vi "Pause_for_server_ch_val.vi"(2 "Extra command string":string, 3 "Simulate/Run":T1) -> (0 "Extra command string Out":string, 1 "Error Comments":string)   [LabVIEW 2010]
uses:
  Controls/User_Specific_mode.ctl
  ADAM Client/Sub VIs/ADAM Controls/Channel_names.ctl
  Globals/Extra_Commands_Global.vi
panel:
  out "Minutes Waited":dbl format="%.2f"
  out "Channel Found?":bool
  out "Time to email next":dbl format="%.2f"
  out "Actual Value":string
  out "Channel Value":string
  out "Channel Name":string
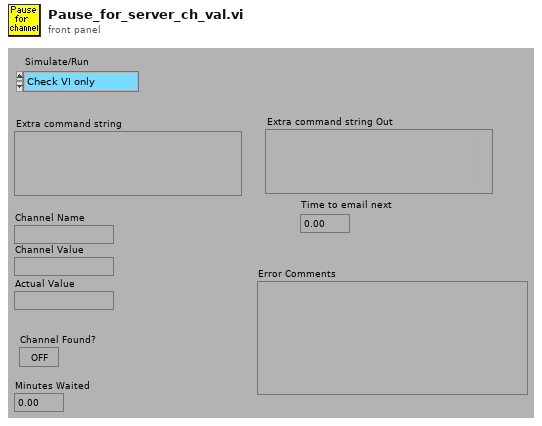
[diagram p1: front panel]
types:
  T1 = typedef "User_Specific_mode.ctl" = enum16{"Check VI only", "Run VI"}
  T2 = typedef "Channel_names.ctl" = enum16{"Active Only", "Active + Off", "All Channels"}
  T3 = typedef "Ch_description_ADAM.ctl" = cluster{"Ch Name":string, "Type":T4, "Function":T5, "Ch State":T6, "Calibration type":T7, "A":dbl, "B":dbl, "C":dbl, "D":dbl, "Comments":string, "Address":T8, "String":string, "Duty":u16}
  T4 = typedef "Module_type_ADAM.ctl" = enum16{"4011", "4012", "4013", "4014", "4016", "4017", "4018", "4021", "4050", "4052", "4053", "4060", "4080", "5000", "5017", "5018", "5024", "5051", "5056", "5060", "6060", "Tracker", "WEST", "GILL", "JEM", "VICI", "Vaisala", "DRUCK", "Run VI Named:", "IR2100", "PPT", "Comparator", "VIRTUAL", "Hold Value", "Read A", "Read Ch", "Coded", "Client Info", "Web Client", "X10", "Test"}
  T5 = typedef "Function_ADAM.ctl" = enum16{"Analogue Input", "Digital Input", "Event counter", "Event rate", "Analogue Output", "Digital Output", "Relay Output"}
  T6 = typedef "Channel_State.ctl" = enum16{"On", "Off", "Always On", "Always Off"}
  T7 = typedef "Calib_type_ADAM.ctl" = enum16{"Raw", "Bx + A", "Cx^2 + Bx + A", "Dx^3 + Cx^2 + Bx + A", "In Band", "Hi-Tec Q", "Hi-Tec M_dot", "Text"}
  T8 = typedef "Address.ctl" = cluster{"Main":i32, "Ch.":i32, "Sub":i32, "Port Name":string}
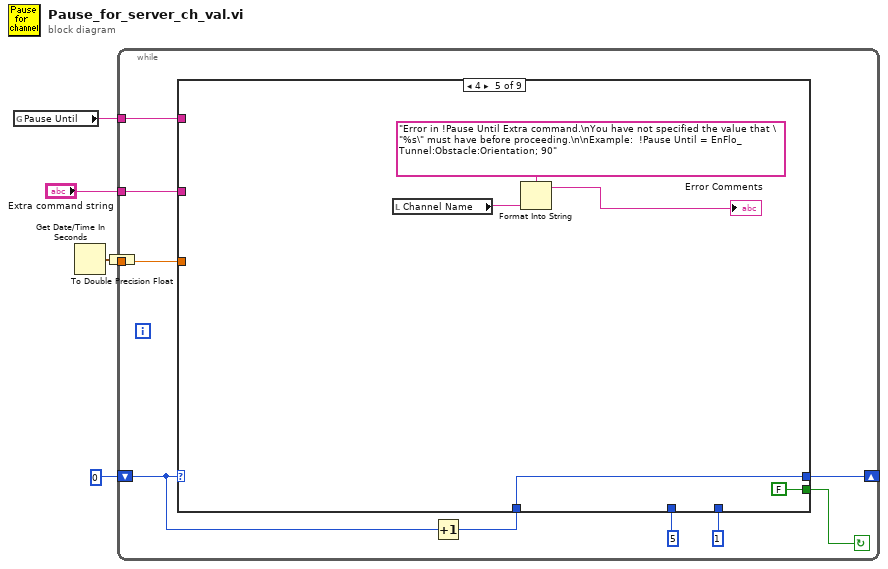
[diagram p0: block diagram]
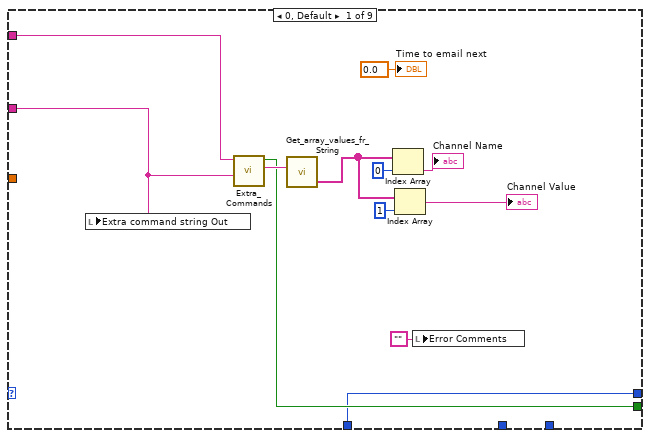
[diagram p2: hidden frame]
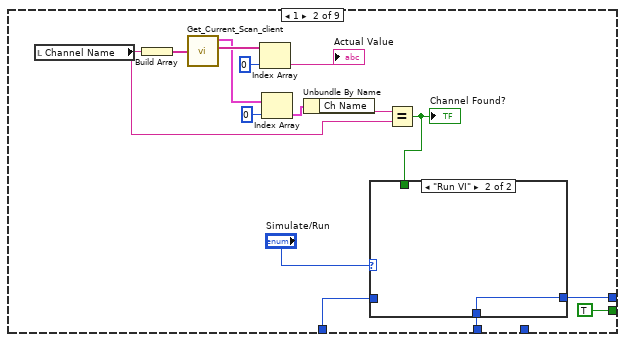
[diagram p3: hidden frame]
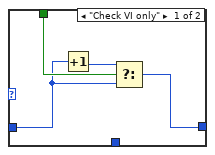
[diagram p4: hidden frame]
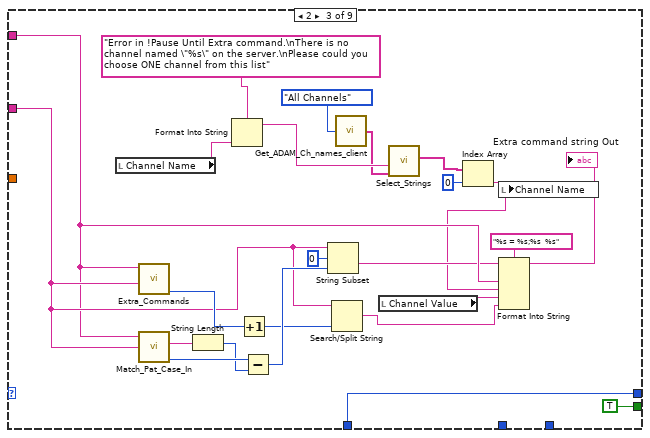
[diagram p5: hidden frame]
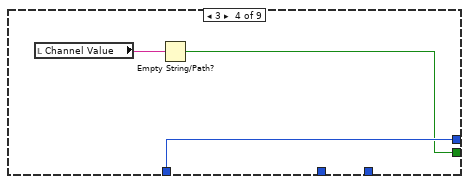
[diagram p6: hidden frame]
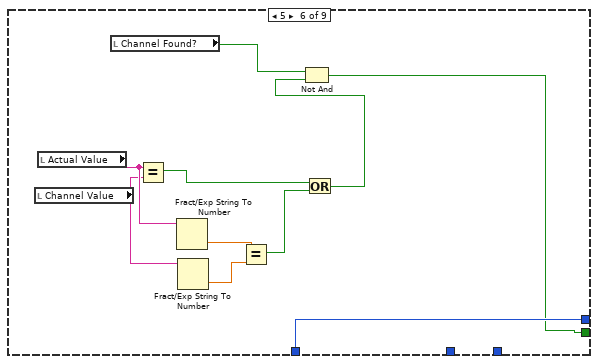
[diagram p7: hidden frame]
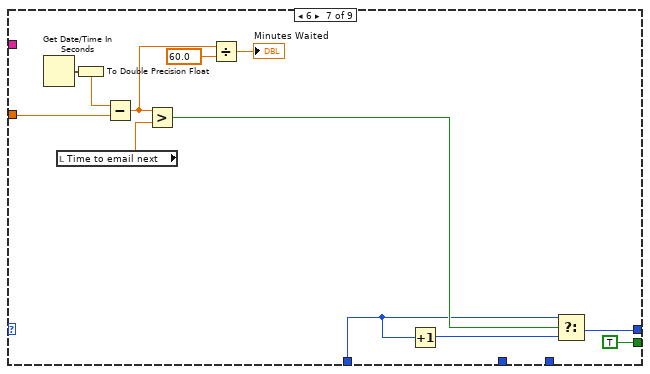
[diagram p8: hidden frame]
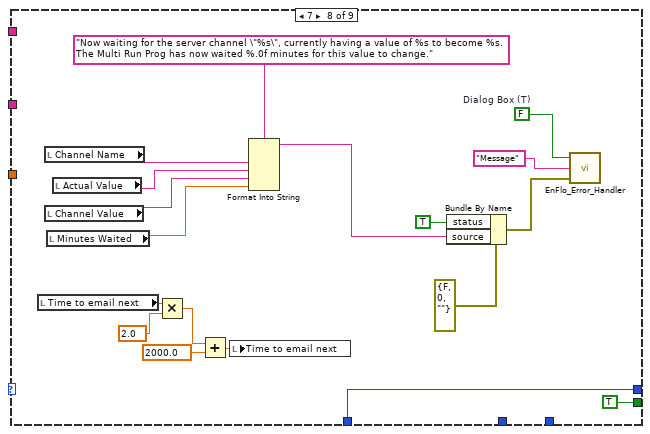
[diagram p9: hidden frame]
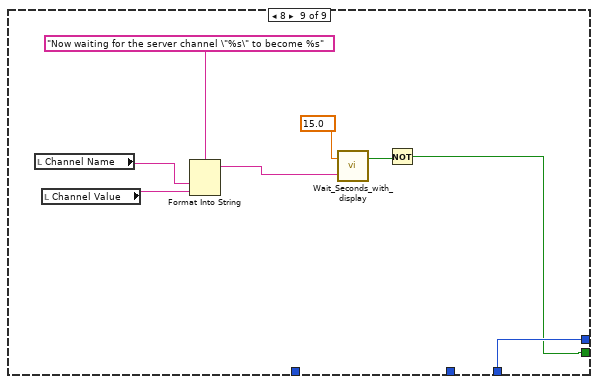
[diagram p10: hidden frame]
diagram:
  n1 = global read "Extra_Commands_Global.vi" "Pause Until"() -> (w3:string)
  n2 = Get Date/Time In Seconds() -> (seconds since 1Jan1904=w1:timestamp)
  n3 = To Double Precision Float(number=w1) -> (double precision float=w2:dbl)
  n4 = while {
    tunnel: w2 -> [w7]
    tunnel: w3 -> [w8]
    tunnel: "Extra command string" -> [w9]
    shift-left: 0 -> [w13]
    shift-right: [w11] -> _
    stop <- w14 continue-if-true
    n5 = Increment(x=w13) -> (x+1=w12:i32)
    n6 = case shown="4" w13 {
      tunnel: [w21 TRUE ("Command Found") TRUE ("Command Found") w71 FALSE ("Command Found") w86 TRUE ("Command Found") TRUE ("Command Found") w119] -> w14
      tunnel: w12 -> [w20 w30 w50 w73 w78 w88 w95 w118 _]
      tunnel: [w20 w29 w50 w73 w78 w88 w93 w118 w121] -> w11
      tunnel: 5 ("f") -> [_ w28 _ _ _ _ _ _ _]
      tunnel: w9 -> [w17 _ w57 _ _ _ _ _ _]
      tunnel: w8 -> [w18 _ w56 _ _ _ _ _ _]
      tunnel: w7 -> [_ _ _ _ _ _ w97 _ _]
      tunnel: 1 ("f") -> [_ _ _ _ _ _ _ _ w121]
      frame 0, Default {
        n7 = local write "Extra command string Out"(w17) -> ()
        n8 = call "Extra_Commands.vi"("String to Search"=w17, "Command"=w18) -> ("String Value"=w26:string, "Command Found"=w21:bool)  [unwired: 1 in, 3 out]
        n9 = call "Get_array_values_fr_String.vi"("String Value"=w26) -> ("String array"=w23:string[])  [unwired: 1 out]
        n10 = Index Array(array=w23, index=0 ("Index")) -> (element=→"Channel Name":string)
        n11 = Index Array(array=w23, index=1 ("Index")) -> (element=→"Channel Value":string)
        n12 = local write "Error Comments"("") -> ()
        "Time to email next" <- 0.0 ("Time to email next")
      }
      frame 1 {
        n13 = local read "Channel Name"() -> (w33:string)
        n14 = Build Array(w33) -> (w41:string[])
        n15 = call "Get_Current_Scan_client.vi"("ADAM Ch Names"=w41) -> ("Ch Description Array"=w37:T3[], "String values"=w40:string[])  [unwired: 2 out]
        n16 = Index Array(array=w40, index=0 ("Index")) -> (element=→"Actual Value":string)
        n17 = Index Array(array=w37, index=0 ("Index")) -> (element=w36:T3)
        n18 = Unbundle By Name(w36) -> ("Ch Name"=w35:string)
        n19 = Equal?(x=w35, y=w33) -> (x = y?=w27:bool)
        "Channel Found?" <- w27
        n20 = case shown="\"Run VI\"" "Simulate/Run" {
          tunnel: w30 -> [w43 _]
          tunnel: [w42 w46] -> w29
          tunnel: w28 -> [_ w46]
          tunnel: w27 -> [w45 _]
          frame "Check VI only" {
            n21 = Increment(x=w43) -> (x+1=w44:i32)
            n22 = Select(t=w44, s=w45, f=w43) -> (s? t:f=w42:i32)
          }
          frame "Run VI" {
          }
        }
      }
      frame 2 {
        n23 = local read "Channel Name"() -> (w68:string)
        n24 = call "Extra_Commands.vi"("String to Search"=w57, "Command"=w56) -> ("Offset Past Command"=w58:i32)  [unwired: 1 in, 4 out]
        n25 = call "Match_Pat_Case_In.vi"("String to match"=w56, "String"=w57) -> ("Matched string"=w63:string, "offset past match"=w62:i32)  [unwired: 1 in, 2 out]
        n26 = String Length(string=w63) -> (length=w61:i32)
        n27 = Format Into String(format string="Error in !Pause Until Extra command.\nThere is no channel named \"%s\" on the server.\nPlease could you choose ONE channel from this list" ("Format String"), w68) -> (resulting string=w67:string)  [unwired: 2 in, 1 out]
        n28 = Increment(x=w58) -> (x+1=w48:i32)
        n29 = Subtract(x=w62, y=w61) -> (x-y=w60:i32)
        n30 = String Subset(string=w57, offset (0)=0, length (rest)=w60) -> (substring=w55:string)
        n31 = Search/Split String(string=w57, offset (0)=w48) -> (match + rest of string=w54:string)  [unwired: 3 out]
        n32 = call "Get_ADAM_Ch_names_client.vi"("Channel names set"=Channel_names."All Channels") -> ("Ch names"=w65:string[])
        n33 = local read "Channel Value"() -> (w51:string)
        n34 = call "Select_Strings.vi"("Available Ch names"=w65, "Message"=w67) -> ("Selected Channel Names"=w47:string[])  [unwired: 2 in, 4 out]
        n35 = Index Array(array=w47, index=0 ("Index")) -> (element=w49:string)
        n36 = local write "Channel Name"(w49) -> ()
        n37 = Format Into String(format string="%s = %s;%s  %s" ("Format String"), initial string=w55, w56, w49, w51, w54) -> (resulting string=→"Extra command string Out":string)  [unwired: 1 in, 1 out]
      }
      frame 3 {
        n38 = local read "Channel Value"() -> (w72:string)
        n39 = Empty String/Path?(string/path=w72) -> (empty?=w71:bool)
      }
      frame 4 {
        n40 = local read "Channel Name"() -> (w74:string)
        n41 = Format Into String(format string="Error in !Pause Until Extra command.\nYou have not specified the value that \"%s\" must have before proceeding.\n\nExample:  !Pause Until = EnFlo_Tunnel:Obstacle:Orientation; 90", w74) -> (resulting string=→"Error Comments":string)  [unwired: 2 in, 1 out]
      }
      frame 5 {
        n42 = local read "Channel Value"() -> (w84:string)
        n43 = local read "Actual Value"() -> (w85:string)
        n44 = local read "Channel Found?"() -> (w87:bool)
        n45 = Equal?(x=w85, y=w84) -> (x = y?=w81:bool)
        n46 = Fract/Exp String To Number(string=w85) -> (number=w83:dbl)  [unwired: 4 out]
        n47 = Fract/Exp String To Number(string=w84) -> (number=w82:dbl)  [unwired: 4 out]
        n48 = Equal?(x=w83, y=w82) -> (x = y?=w80:bool)
        n49 = Or(x=w81, y=w80) -> (x .or. y?=w79:bool)
        n50 = Not And(1:w79, 2:w87) -> (0:w86:bool)
      }
      frame 6 {
        n51 = Get Date/Time In Seconds() -> (seconds since 1Jan1904=w89:timestamp)
        n52 = local read "Time to email next"() -> (w98:dbl)
        n53 = To Double Precision Float(number=w89) -> (double precision float=w99:dbl)
        n54 = Subtract(x=w99, y=w97) -> (x-y=w92:dbl)
        n55 = Greater?(x=w92, y=w98) -> (0:w96:bool)
        n56 = Divide(x=w92, y=60.0) -> (x/y=→"Minutes Waited":dbl)
        n57 = Increment(x=w95) -> (x+1=w94:i32)
        n58 = Select(t=w95, s=w96, f=w94) -> (s? t:f=w93:i32)
      }
      frame 7 {
        w114 = FALSE  # Dialog Box (T)
        n59 = local read "Time to email next"() -> (w105:dbl)
        n60 = local read "Channel Name"() -> (w113:string)
        n61 = local read "Channel Value"() -> (w111:string)
        n62 = local read "Minutes Waited"() -> (w110:dbl)
        n63 = local read "Actual Value"() -> (w112:string)
        n64 = Multiply(x=w105, y=2.0) -> (x*y=w103:dbl)
        n65 = Add(x=w103, y=2000.0) -> (x+y=w101:dbl)
        n66 = local write "Time to email next"(w101) -> ()
        n67 = Format Into String(format string="Now waiting for the server channel \"%s\", currently having a value of %s to become %s. The Multi Run Prog has now waited %.0f minutes for this value to change." ("Format String"), w113, w112, w111, w110) -> (resulting string=w106:string)  [unwired: 2 in, 1 out]
        n68 = Bundle By Name(cluster=errorcluster {"status"=FALSE, "code"=0, "source"=""} ("error in (no error)"), "status"=TRUE ("Bundle Element"), "source"=w106) -> (w115:errorcluster)
        n69 = call "EnFlo_Error_Handler.vi"("error in (no error)"=w115, "Error Type"="Message", "Dialog Box (T)"=w114) -> ()  [unwired: 3 out]
      }
      frame 8 {
        n70 = local read "Channel Name"() -> (w125:string)
        n71 = local read "Channel Value"() -> (w124:string)
        n72 = Format Into String(format string="Now waiting for the server channel \"%s\" to become %s" ("Format String"), w125, w124) -> (resulting string=w122:string)  [unwired: 2 in, 1 out]
        n73 = call "Wait_Seconds_with_display.vi"("Message"=w122, "Seconds to wait"=15.0) -> ("Stopped"=w120:bool)  [unwired: 1 out]
        n74 = Not(x=w120) -> (.not. x?=w119:bool)
      }
    }
  }
